vi "Set AVG Mode Frame Num.vi"(8 "error in (no error)":errorcluster, 10 "nFrameNum":i32, 11 "nSensorIP":u32) -> (0 "error out":errorcluster, 3 "function return":i32)   [LabVIEW 2017, in "imgAcquisition.lvlib"]
doc: "DLLFunction int __stdcall ImageCapSetAVGModeFrameNum(unsigned int nSensorIP, int nFrameNum);"
uses:
  imgAcquisition.lvlib
  lib/ImageCaptureDLL.dll
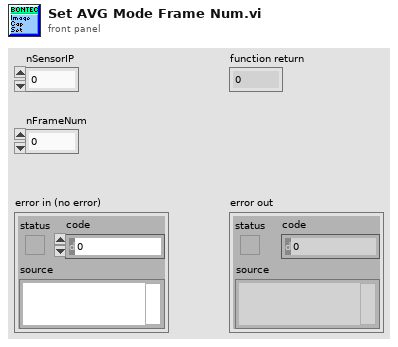
[diagram p1: front panel]
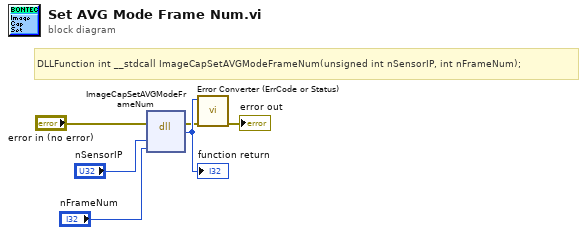
[diagram p0: block diagram]
diagram:
  # "DLLFunction int __stdcall ImageCapSetAVGModeFrameNum(unsigned int nSensorIP, int nFrameNum);"
  n1 = dll-call lib="F:/BonTechFlatPanelLVDriver/lib/ImageCaptureDLL.*" fn="ImageCapSetAVGModeFrameNum"(error in="error in (no error)", "nSensorIP"="nSensorIP", "nFrameNum"="nFrameNum") -> (error out=w2:errorcluster, w6:i32)  [unwired: 4 in, 1 out]
  "function return" <- w6
  n2 = call "Error Converter (ErrCode or Status).vi"("error in (no error)"=w2, "error code"=w6) -> ("error out"=→"error out":errorcluster)  [unwired: 9 in]
